vi "AVTCP-Delete Files.vi"(0 "Folder":string, 7 "Pattern":string) -> (15 "error out":errorcluster)   [LabVIEW 2020]
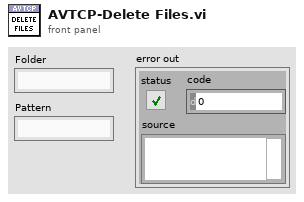
[diagram p1: front panel]
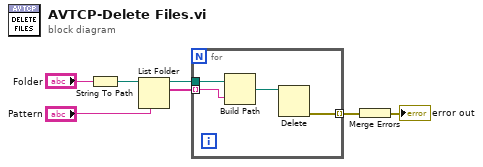
[diagram p0: block diagram]
diagram:
  n1 = String To Path(string="Folder") -> (path=w3:path)
  n2 = List Folder(path=w3, pattern="Pattern") -> (path out=w7:path, filenames=w6:string[])  [unwired: 2 in, 2 out]
  n3 = for {
    tunnel: w7 -> [w11]
    tunnel: w6 -> [w10] mode=indexing
    tunnel: [w8] -> w5 mode=indexing
    n4 = Build Path(base path=w11, name or relative path=w10) -> (appended path=w9:path)
    n5 = Delete(path (use dialog)=w9) -> (error out=w8:errorcluster)  [unwired: 4 in, 2 out]
  }
  n6 = Merge Errors(w5) -> (→"error out":errorcluster)
